vi "Close NI-DMM Session.vi"(8 "error in (no error)":errorcluster, 10 "session information":T1, 11 "instrument handle":refnum<k15>) -> (0 "error out":errorcluster)   [LabVIEW 2020, in "NIDMM.lvlib"]
doc: "Closes the given NI-DCPower instrument handle."
uses:
  NIDMM.lvlib
  <vilib>/MeasurementLink/MeasurementLink Session Management Client/RPC Messages/ni_measurementlink_sessionmanagement_v1_SessionInformation.ctl
  <vilib>/MeasurementLink/MeasurementLink Session Management Client/RPC Messages/nidevice_grpc_Session.ctl
  <vilib>/MeasurementLink/MeasurementLink Session Management Client/RPC Messages/ni_measurementlink_sessionmanagement_v1_ChannelMapping.ctl
  <vilib>/MeasurementLink/MeasurementLink Session Management Client/MeasurementLink Session Management Client.lvlib
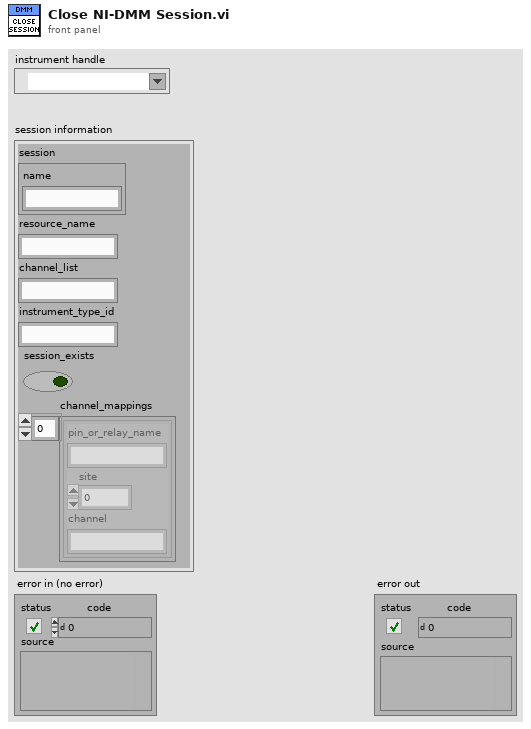
[diagram p1: front panel]
types:
  T1 = typedef "MeasurementLink Session Management Client.lvlib/ni_measurementlink_sessionmanagement_v1_SessionInformation.ctl" = cluster{"session":T2, "resource_name":string, "channel_list":string, "instrument_type_id":string, "session_exists":bool, "channel_mappings":T3[]}
  T2 = typedef "MeasurementLink Session Management Client.lvlib/nidevice_grpc_Session.ctl" = cluster{"name":string}
  T3 = typedef "MeasurementLink Session Management Client.lvlib/ni_measurementlink_sessionmanagement_v1_ChannelMapping.ctl" = cluster{"pin_or_relay_name":string, "site":i32, "channel":string}
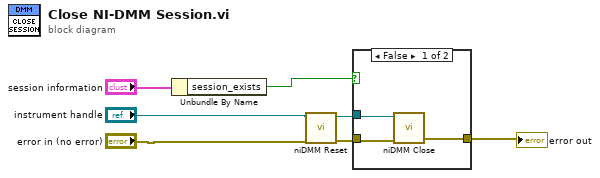
[diagram p0: block diagram]
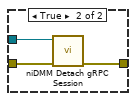
[diagram p2: hidden frame]
diagram:
  n1 = Unbundle By Name("session information") -> ("session_exists"=w5:bool)
  n2 = call <instrlib>:"niDMM Reset.vi"("error in (no error)"="error in (no error)", "instrument handle"="instrument handle") -> ("error out"=w4:errorcluster, "instrument handle out"=w3:refnum<k15>)  [unwired: 8 in]
  n3 = case shown="False" w5 {
    tunnel: w3 -> [w10 w11]
    tunnel: w4 -> [w9 w12]
    tunnel: [w8 w13] -> w6
    frame False {
      n4 = call <instrlib>:"niDMM Close.vi"("error in (no error)"=w9, "instrument handle"=w10) -> ("error out"=w8:errorcluster)  [unwired: 9 in]
    }
    frame True {
      n5 = call <instrlib>:"niDMM Detach gRPC Session.vi"("error in (no error)"=w12, "instrument handle"=w11) -> ("error out"=w13:errorcluster)  [unwired: 9 in]
    }
  }
  "error out" <- w6
